vi "Replace Outside Items.vi"(0 "shared directory":path, 5 "outside vis":string[](array[string]), 7 "dependent vis":path[](array[path]), 9 "measurement directory":path, 11 "error in":errorcluster) -> (15 "error out":errorcluster)   [LabVIEW 2021, in "Multiple Converter.lvlib"]
uses:
  Multiple Converter.lvlib
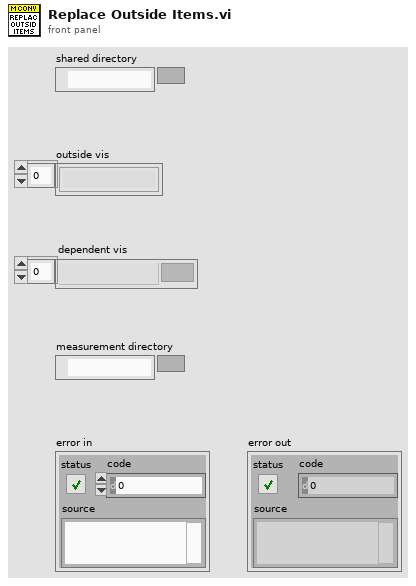
[diagram p1: front panel]
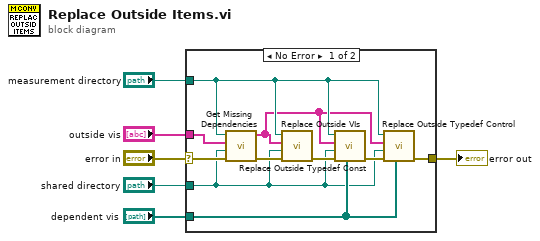
[diagram p0: block diagram]
diagram:
  n1 = case shown="No Error" "error in" {
    selector: "error in" -> [w14 w17]
    tunnel: "outside vis" -> [w13 _]
    tunnel: [w12 w17] -> w5
    tunnel: "measurement directory" -> [w9 _]
    tunnel: "shared directory" -> [w7 _]
    tunnel: "dependent vis" -> [w10 _]
    frame No Error {
      n2 = call "Get Missing Dependencies.vi"("error in"=w14, "shared directory"=w7, "outside vis in"=w13, "measurement directory"=w9) -> ("error out"=w15:errorcluster, "outside vis out"=w8:string[])  [unwired: 6 in]
      n3 = call "Replace Outside VIs.vi"("error in (no error)"=w15, "Shared directory"=w7, "Non-Library VI[]"=w8, "Measurement directory"=w9) -> ("error out"=w16:errorcluster)  [unwired: 7 in]
      n4 = call "Replace Outside Typedef Const.vi"("Dependent VIs"=w10, "error in (no error)"=w16, "Shared directory"=w7, "Non-Library VI[]"=w8, "Measurement Directory"=w9) -> ("error out"=w11:errorcluster)  [unwired: 6 in]
      n5 = call "Replace Outside Typedef Control.vi"("Dependent VIs"=w10, "error in (no error)"=w11, "Shared directory"=w7, "Non-Library VI[]"=w8, "Measurement Directory"=w9) -> ("error out"=w12:errorcluster)  [unwired: 6 in]
    }
    frame Error {
    }
  }
  "error out" <- w5
